vi "TrioMotion Controller.vi"(10 "Notifiers":T2, 11 "Channel in":T1) -> (3 "channel out":T1)   [LabVIEW 2020, in "TrioMotion Controller.lvlib"]
uses:
  TrioMotion Controller.lvlib
  <extravilib>/ChannelInstances/Messenger-t'Message Queue.lvlib-Message Cluster.ctl'/))Channel.ctl
  support/Message Queue/Message Cluster.ctl
  support/Notifiers/Notifiers.ctl
  TrioData.ctl
  Connection Type.ctl
  Axis Parameters.ctl
  controls/MHL Data.ctl
  controls/MHL UI Data.ctl
  controls/MHL Status.ctl
  controls/MHL References.ctl
  controls/MHL Configuration.ctl
  support/SR-Test Med System Globals.vi
  <vilib>/Utility/error.llb/Error Cluster From Error Code.vi
  <vilib>/ErrorRing/Error Ring.xnode
  support/Message Queue/Message Queue.lvlib
  <extravilib>/ChannelInstances/Messenger-t'Message Queue.lvlib-Message Cluster.ctl'.lvlib
panel:
  in  "TrioPC":refnum<k7>(container)
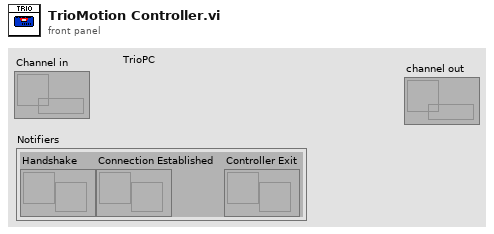
[diagram p1: front panel]
types:
  T1 = typedef "Messenger-t'Message Queue.lvlib-Message Cluster.ctl'.lvlib/))Channel.ctl" = refnum<queue>
  T2 = typedef "Notifiers.ctl" = cluster{"Handshake":refnum<notifier>, "Connection Established":refnum<notifier>, "Controller Exit":refnum<notifier>}
  T3 = typedef "TrioMotion Controller.lvlib/TrioData.ctl" = cluster{"Connected":bool, "Connection Method":T4, "Product Name":string, " Version":string, "Controller Type":string, "SerialCommPort":fxp<+,3,3>, "Programs List":string[], "X Axis Parameters":T5, "A Axis Parameters":T5}
  T4 = typedef "TrioMotion Controller.lvlib/Connection Type.ctl" = enum16{"USB", "Serial", "Ethernet", "PCI", "Path", "No connection"}
  T5 = typedef "TrioMotion Controller.lvlib/Axis Parameters.ctl" = cluster{"ATYPE":dbl, "P_GAIN":dbl, "I_GAIN":dbl, "D_GAIN":dbl, "0V_GAIN":dbl, "VFF_GAIN":dbl, "UNITS":dbl, "SPEED":dbl, "ACCEL":dbl, "DECEL":dbl, "CREEP":dbl, "JOGSPEED":dbl, "FE_LIMIT":dbl, "DAC":dbl, "SERVO":dbl, "REP_DIST":dbl, "FWD_IN":dbl, "REV_IN":dbl, "DATUM_IN":dbl, "FH_IN":dbl, "FS_LIMIT":dbl, "RS_LIMIT":dbl, "MTYPE":dbl, "NTYPE":dbl, "MPOS":dbl, "FE":dbl, "AXISSTATUS":dbl, "VPSPEED":dbl}
  T6 = enum16{"open", "replace", "create", "open or create", "replace or create", "replace or create with confirmation"}
  T7 = typedef "MHL Data.ctl" = cluster{"MHL UI Data":T8, "MHL References":T10, "MHL Configuration":T11}
  T8 = typedef "MHL UI Data.ctl" = cluster{"Status":string, "Connection Type":T4, "Connected to Controller":bool, "Axes Enabled":bool, "Jogging Enabled":bool, "X Axis MPOS":dbl, "A Axis MPOS":dbl, "X Axis SPEED":dbl, "A Axis SPEED":dbl, "Plot Laser Data":bool, "MHL Status":T9}
  T9 = typedef "MHL Status.ctl" = enum16{"Disconnected", "Connecting", "Connected", "Axes Enabled", "Machine Running", "Shutdown"}
  T10 = typedef "MHL References.ctl" = cluster{"Connect to Controller Ref":refnum<vi>, "Connection Type Ref":refnum<vi>, "Set Parameters Ref":refnum<vi>, "Enable Axes Ref":refnum<vi>, "Home Axes Ref":refnum<vi>}
  T11 = typedef "MHL Configuration.ctl" = cluster{"Fuel Control Valve Maximum":dbl, "Fuel Control Valve Minimum":dbl}
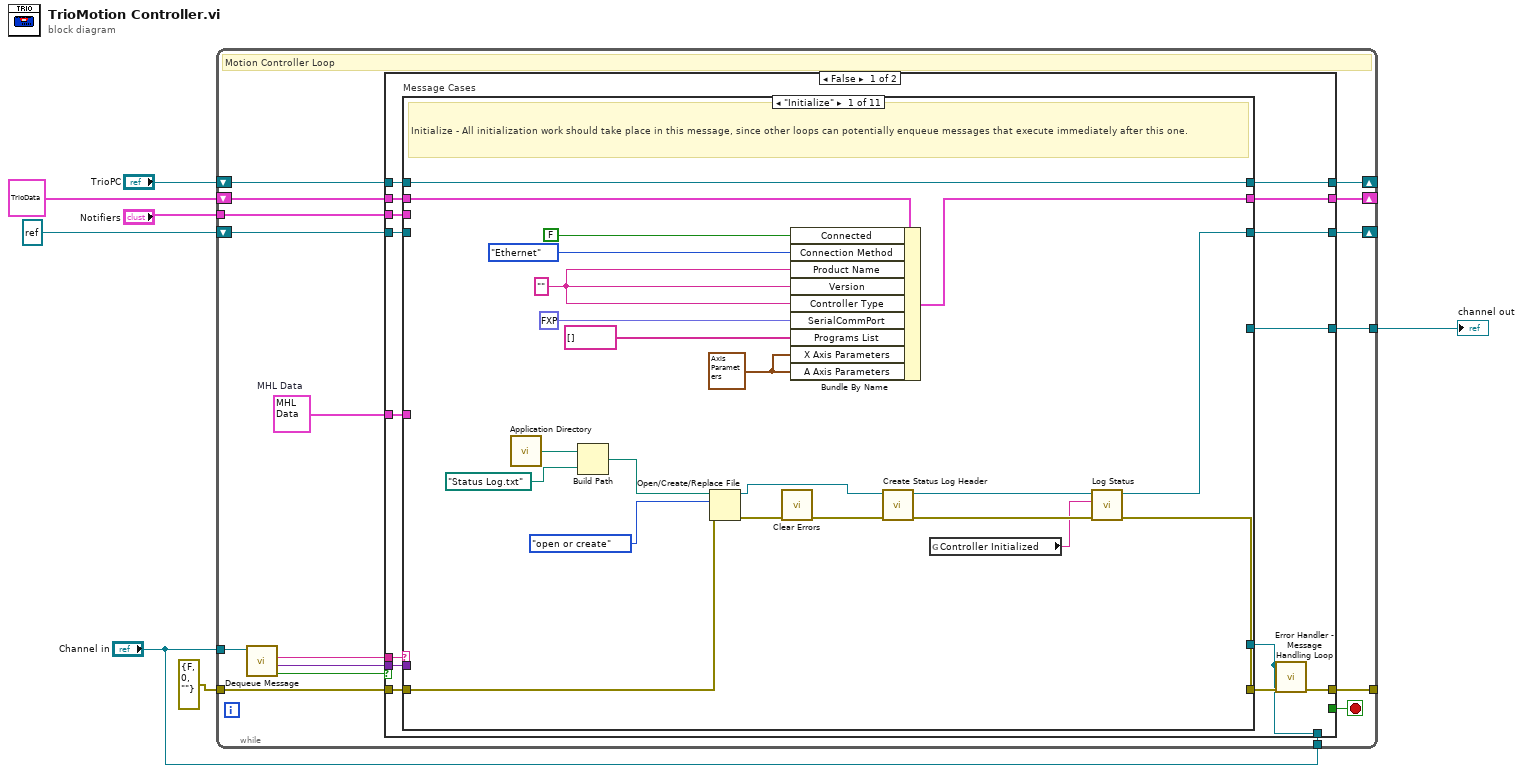
[diagram p0: block diagram]
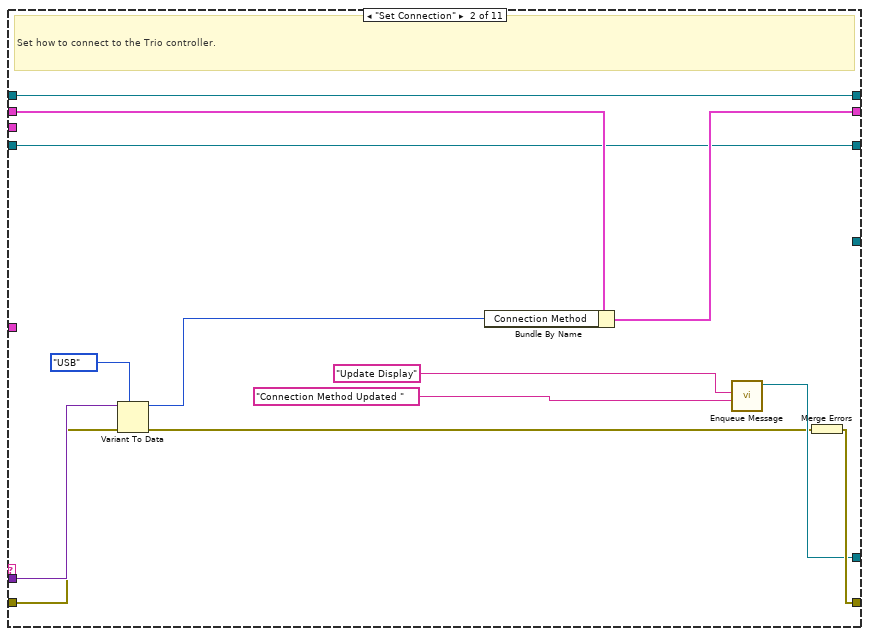
[diagram p2: hidden frame]
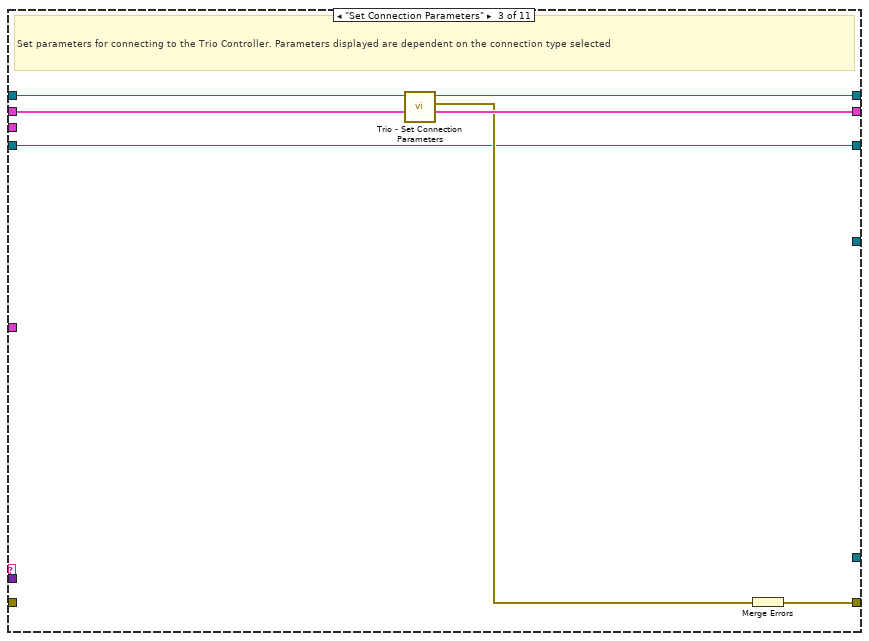
[diagram p3: hidden frame]
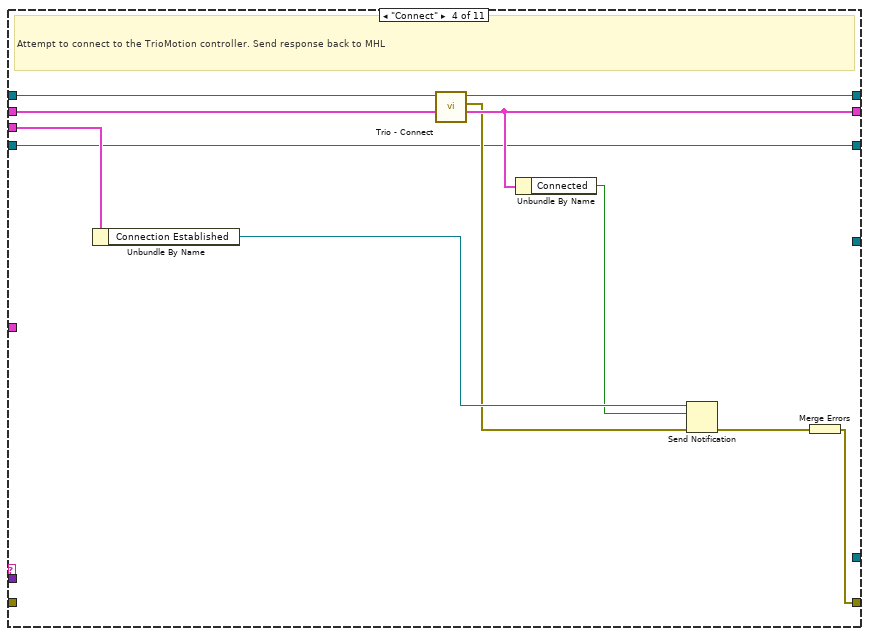
[diagram p4: hidden frame]
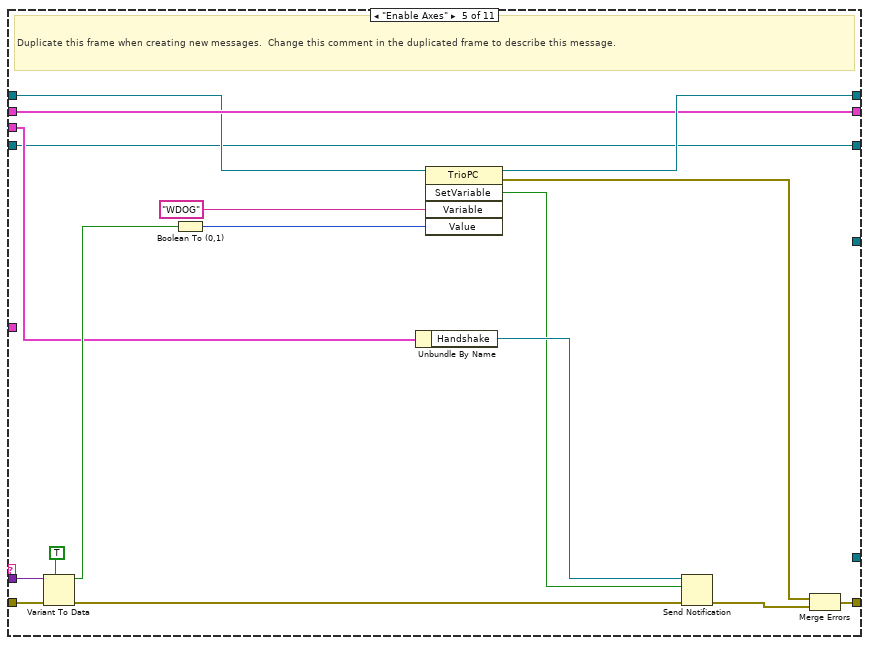
[diagram p5: hidden frame]
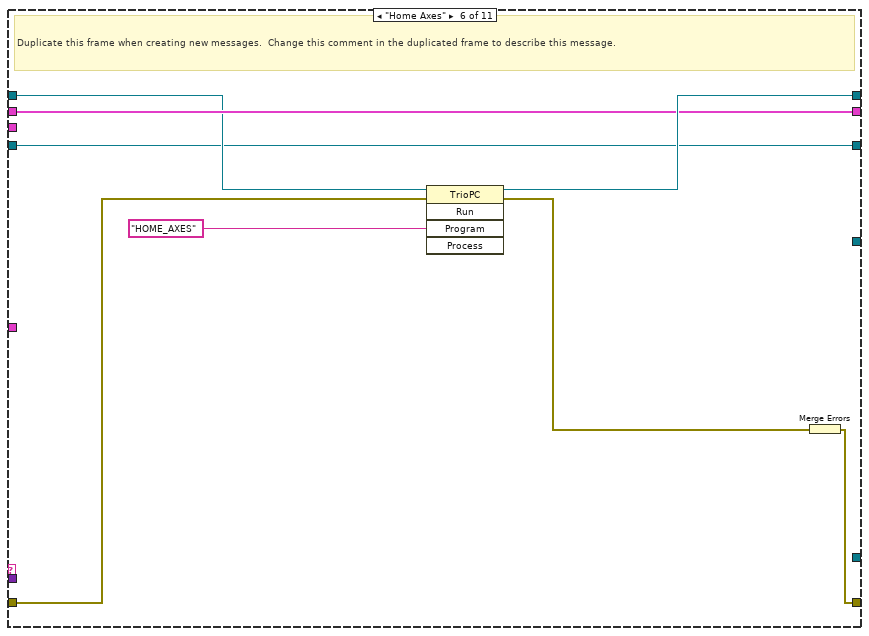
[diagram p6: hidden frame]
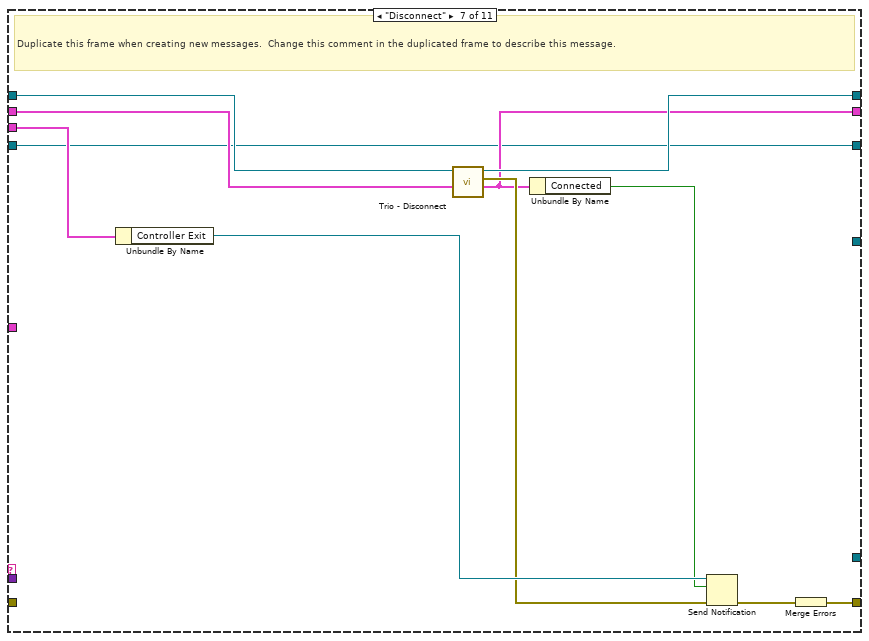
[diagram p7: hidden frame]
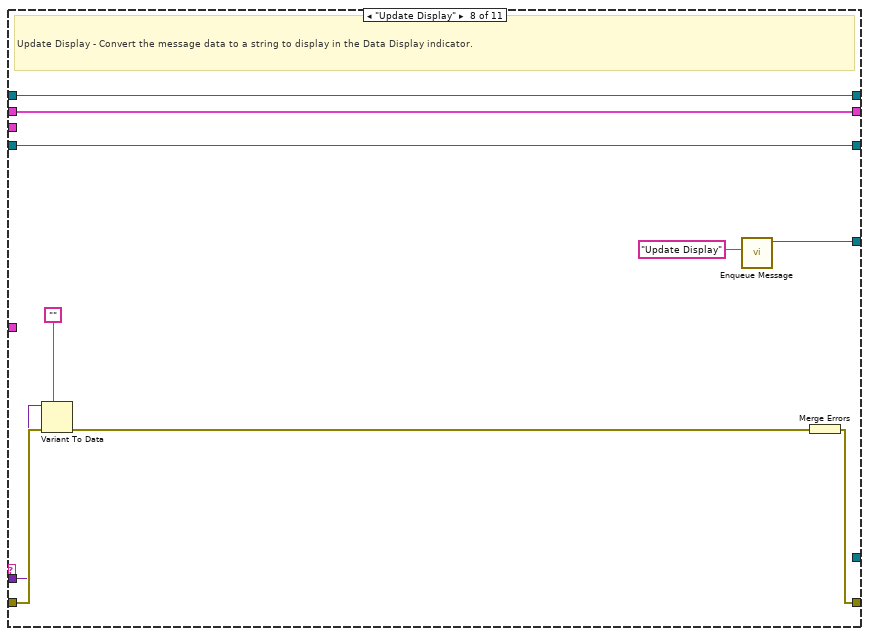
[diagram p8: hidden frame]
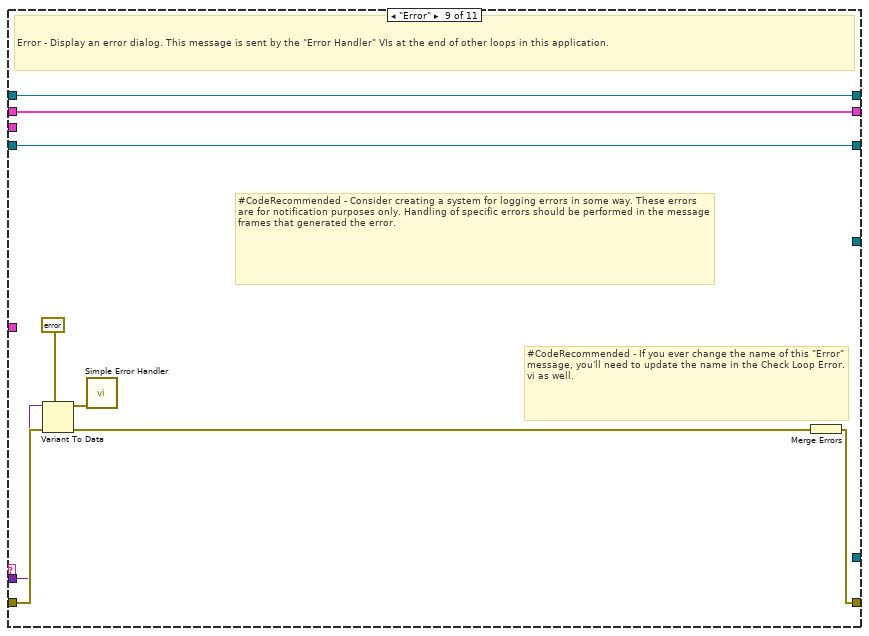
[diagram p9: hidden frame]
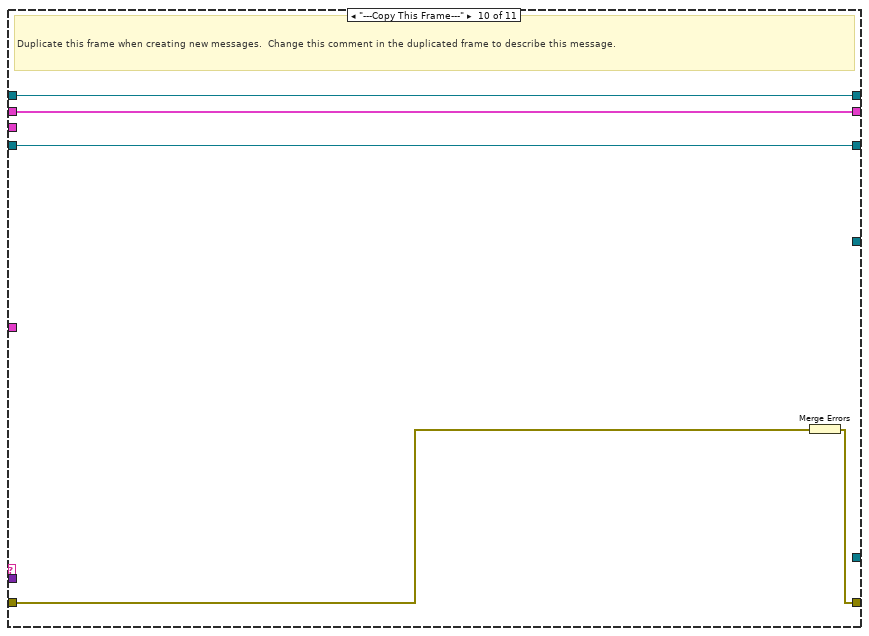
[diagram p10: hidden frame]
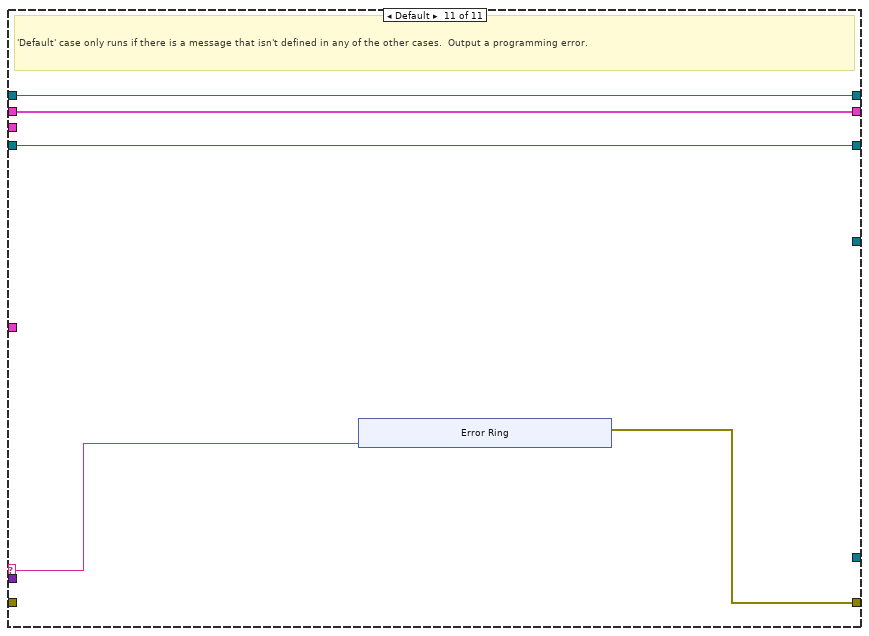
[diagram p11: hidden frame]
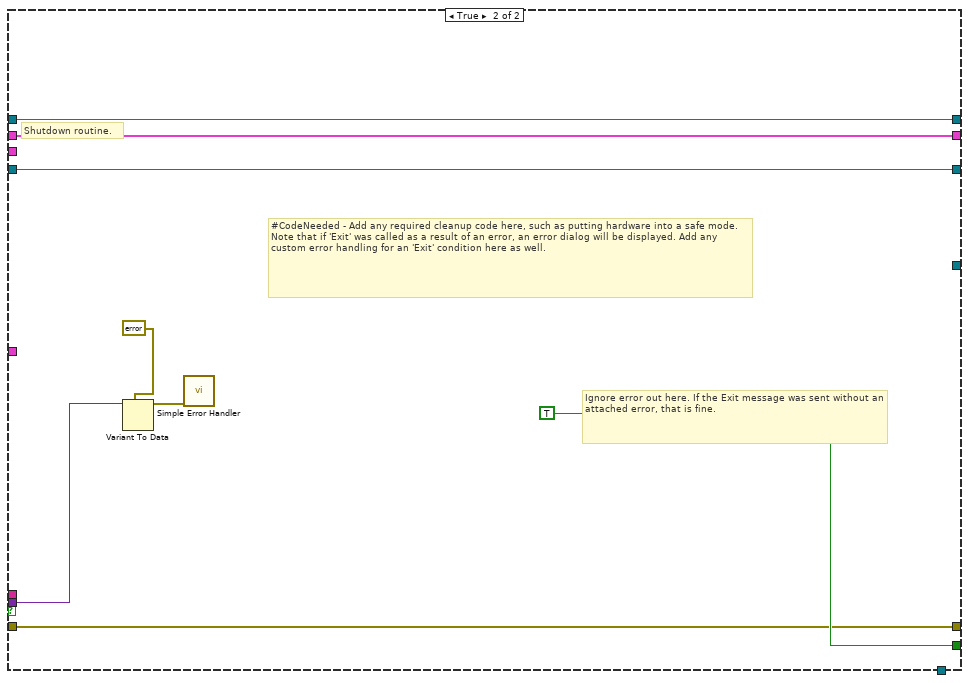
[diagram p12: hidden frame]
diagram:
  n1 = while {
    shift-right: [w23] -> _
    shift-left: T3 {"Connected"=FALSE, "Connection Method"=enum."USB", "Product Name"="", " Version"="", "Controller Type"="", "SerialCommPort"=0.0, "Programs List"=[], "X Axis Parameters"={"ATYPE"=0.0, "P_GAIN"=0.0, "I_GAIN"=0.0, "D_GAIN"=0.0, "0V_GAIN"=0.0, "VFF_GAIN"=0.0, "UNITS"=0.0, "SPEED"=0.0, "ACCEL"=0.0, "DECEL"=0.0, "CREEP"=0.0, "JOGSPEED"=0.0, "FE_LIMIT"=0.0, "DAC"=0.0, "SERVO"=0.0, "REP_DIST"=0.0, "FWD_IN"=0.0, "REV_IN"=0.0, "DATUM_IN"=0.0, "FH_IN"=0.0, "FS_LIMIT"=0.0, "RS_LIMIT"=0.0, "MTYPE"=0.0, "NTYPE"=0.0, "MPOS"=0.0, "FE"=0.0, "AXISSTATUS"=0.0, "VPSPEED"=0.0}, "A Axis Parameters"={"ATYPE"=0.0, "P_GAIN"=0.0, "I_GAIN"=0.0, "D_GAIN"=0.0, "0V_GAIN"=0.0, "VFF_GAIN"=0.0, "UNITS"=0.0, "SPEED"=0.0, "ACCEL"=0.0, "DECEL"=0.0, "CREEP"=0.0, "JOGSPEED"=0.0, "FE_LIMIT"=0.0, "DAC"=0.0, "SERVO"=0.0, "REP_DIST"=0.0, "FWD_IN"=0.0, "REV_IN"=0.0, "DATUM_IN"=0.0, "FH_IN"=0.0, "FS_LIMIT"=0.0, "RS_LIMIT"=0.0, "MTYPE"=0.0, "NTYPE"=0.0, "MPOS"=0.0, "FE"=0.0, "AXISSTATUS"=0.0, "VPSPEED"=0.0}} ("TrioData") -> [w24]
    tunnel: [w21] -> _
    tunnel: "Channel in" -> [w18]
    tunnel: errorcluster {"status"=FALSE, "code"=0, "source"=""} ("error IO") -> [w20]
    tunnel: "Channel in" -> [w19]
    shift-right: [w13] -> _
    shift-left: "TrioPC" -> [w14]
    tunnel: "Notifiers" -> [w12]
    tunnel: [w11] -> w3
    shift-right: [w8] -> _
    shift-left: refnum<file> refnum ("Log File Refnum Out") -> [w9]
    stop <- w22 stop-if-true
    w10 = T7 {"MHL UI Data"={"Status"="", "Connection Type"=enum."Ethernet", "Connected to Controller"=FALSE, "Axes Enabled"=FALSE, "Jogging Enabled"=FALSE, "X Axis MPOS"=0.0, "A Axis MPOS"=0.0, "X Axis SPEED"=0.0, "A Axis SPEED"=0.0, "Plot Laser Data"=FALSE, "MHL Status"=enum."Disconnected"}, "MHL References"={"Connect to Controller Ref"=refnum, "Connection Type Ref"=refnum, "Set Parameters Ref"=refnum, "Enable Axes Ref"=refnum, "Home Axes Ref"=refnum}, "MHL Configuration"={"Fuel Control Valve Maximum"=0.0, "Fuel Control Valve Minimum"=0.0}}  # MHL Data
    # "Motion Controller Loop"
    n2 = call "Dequeue Message.vi"("channel"=w18) -> ("channel aborted"=w15:bool, "message data"=w16:variant, "message"=w17:string)  [unwired: 8 in]
    n3 = case shown="False" w15 {
      tunnel: w24 -> [w39 w170]
      tunnel: [w38 w170] -> w23
      tunnel: [_ TRUE] -> w22
      tunnel: [w37 w171] -> w21
      tunnel: w17 -> [w35 _]
      tunnel: w16 -> [w34 w167]
      tunnel: w20 -> [w33 w171]
      tunnel: [w32 _] -> w19
      tunnel: w14 -> [w31 w166]
      tunnel: [w30 w166] -> w13
      tunnel: w12 -> [w29 _]
      tunnel: [w28 _] -> w11
      tunnel: w10 -> [w27 _]
      tunnel: w9 -> [w26 w165]
      tunnel: [w25 w165] -> w8
      frame False {
        n4 = case "Message Cases" shown="\"Initialize\"" w35 {
          selector: w35 -> [_ _ _ _ _ _ _ _ _ _ w155]
          tunnel: w33 -> [w47 w66 _ _ w103 w111 _ w136 w147 w152 _]
          tunnel: [w40 w74 w81 w92 w109 w117 w128 w137 w141 w150 w156] -> w36
          tunnel: w39 -> [w61 w69 w80 w89 w107 w115 w125 w138 w146 w151 w157]
          tunnel: [w60 w67 w79 w88 w107 w115 w121 w138 w146 w151 w157] -> w38
          tunnel: w34 -> [_ w68 _ _ w102 _ _ w135 w145 _ _]
          tunnel: [_ w73 _ _ _ _ _ _ _ _ _] -> w32
          tunnel: w31 -> [w56 w64 w78 w91 w106 w114 w127 w132 w140 w149 w154]
          tunnel: [w56 w64 w77 w90 w108 w116 w126 w132 w140 w149 w154] -> w30
          tunnel: w29 -> [_ _ _ w87 w99 _ w123 _ _ _ _]
          tunnel: [_ _ _ _ _ _ _ w131 _ _ _] -> w28
          tunnel: w27 -> [_ _ _ _ _ _ _ _ _ _ _]
          tunnel: w26 -> [_ w62 w75 w82 w93 w110 w118 w129 w139 w148 w153]
          tunnel: [w41 w62 w75 w82 w93 w110 w118 w129 w139 w148 w153] -> w25
          frame "Initialize" {
            w53 = T5 {"ATYPE"=0.0, "P_GAIN"=0.0, "I_GAIN"=0.0, "D_GAIN"=0.0, "0V_GAIN"=0.0, "VFF_GAIN"=0.0, "UNITS"=0.0, "SPEED"=0.0, "ACCEL"=0.0, "DECEL"=0.0, "CREEP"=0.0, "JOGSPEED"=0.0, "FE_LIMIT"=0.0, "DAC"=0.0, "SERVO"=0.0, "REP_DIST"=0.0, "FWD_IN"=0.0, "REV_IN"=0.0, "DATUM_IN"=0.0, "FH_IN"=0.0, "FS_LIMIT"=0.0, "RS_LIMIT"=0.0, "MTYPE"=0.0, "NTYPE"=0.0, "MPOS"=0.0, "FE"=0.0, "AXISSTATUS"=0.0, "VPSPEED"=0.0} ("X Axis Parameters")
            w55 = "" ("Product Name")
            # "Initialize - All initialization work should take place in this message, since other loops can potentially enqueue messages that execute immediately after this one."
            n5 = call <vilib>:"Application Directory.vi"() -> ("Application Directory"=w52:path)
            n6 = Build Path(base path=w52, name or relative path=path "Status Log.txt") -> (appended path=w50:path)
            n7 = Open/Create/Replace File(file path (use dialog)=w50, error in=w47, operation (0:open)=T6."open or create") -> (refnum out=w45:refnum<file>, error out=w48:errorcluster)  [unwired: 3 in, 1 out]
            n8 = call <vilib>:"Clear Errors.vi"("error in (no error)"=w48) -> ("error out"=w46:errorcluster)  [unwired: 5 in, 1 out]
            n9 = Bundle By Name(cluster=w61, "Connected"=FALSE, "Connection Method"=Connection_Type."Ethernet", "Product Name"=w55, "Version"=w55, "Controller Type"=w55, "SerialCommPort"=fxp<+,3,3> 0.0, "Programs List"=string[] [], "X Axis Parameters"=w53, "A Axis Parameters"=w53) -> (w60:T3)
            n10 = call "Create Status Log Header.vi"("error in"=w46, "Log File Refnum in"=w45) -> ("error out"=w44:errorcluster, "Log File Refnum out"=w43:refnum<file>)  [unwired: 8 in]
            n11 = global read "SR-Test Med System Globals.vi" "Controller Initialized"() -> (w42:string)
            n12 = call "Log Status.vi"("error in"=w44, "Event String"=w42, "Log File Refnum In"=w43) -> ("error out"=w40:errorcluster, "Log File Refnum Out"=w41:refnum<file>)  [unwired: 7 in]
          }
          frame "Set Connection" {
            # "Set how to connect to the Trio controller."
            n13 = Variant To Data(error in=w66, type=Connection_Type."USB" ("Connection Method"), Variant=w68) -> (data=w70:T4, error out=w65:errorcluster)
            n14 = Bundle By Name(cluster=w69, "Connection Method"=w70) -> (w67:T3)
            n15 = call "Enqueue Message.vi"("data (empty)"="Connection Method Updated " ("\"Do Something\" button pressed"), "message"="Update Display" ("Message")) -> ("channel"=w73:T1)  [unwired: 9 in]
            n16 = Merge Errors(w65) -> (w74:errorcluster)
          }
          frame "Set Connection Parameters" {
            # "Set parameters for connecting to the Trio Controller. Parameters displayed are dependent on the connection type selected"
            n17 = call "Trio - Set Connection Parameters.vi"("TrioData In"=w80, "TrioControl Refnum in"=w78) -> ("TrioData Out"=w79:T3, "error out"=w76:errorcluster, "TrioControl Refnum Out"=w77:refnum<k7>)  [unwired: 7 in]
            n18 = Merge Errors(w76) -> (w81:errorcluster)
          }
          frame "Connect" {
            # "Attempt to connect to the TrioMotion controller. Send response back to MHL"
            n19 = Unbundle By Name(w87) -> ("Connection Established"=w86:refnum<notifier>)
            n20 = call "Trio - Connect.vi"("TrioData In"=w89, "Trio Reference In"=w91) -> ("TrioData Out"=w88:T3, "error out"=w83:errorcluster, "Trio Reference Out"=w90:refnum<k7>)  [unwired: 7 in]
            n21 = Unbundle By Name(w88) -> ("Connected"=w85:bool)
            n22 = Send Notification(notification=w85, notifier=w86, error in (no error)=w83) -> (error out=w84:errorcluster)  [unwired: 1 out]
            n23 = Merge Errors(w84) -> (w92:errorcluster)
          }
          frame "Enable Axes" {
            # "Duplicate this frame when creating new messages.  Change this comment in the duplicated frame to describe this message."
            n24 = Variant To Data(error in=w103, type=TRUE, Variant=w102) -> (data=w101:bool, error out=w94:errorcluster)
            n25 = Boolean To (0,1)(Boolean=w101) -> (0, 1=w100:i16)
            n26 = Unbundle By Name(w99) -> ("Handshake"=w98:refnum<notifier>)
            n27 = invoke class="TrioPC" method="SetVariable"(reference=w106, "Variable"="WDOG", "Value"=w100) -> (reference out=w108:refnum<k7>, error out=w95:errorcluster, "SetVariable"=w97:bool)  [unwired: 2 in, 2 out]
            n28 = Send Notification(notification=w97, notifier=w98, error in (no error)=w94) -> (error out=w96:errorcluster)  [unwired: 1 out]
            n29 = Merge Errors(w95, w96) -> (w109:errorcluster)
          }
          frame "Home Axes" {
            # "Duplicate this frame when creating new messages.  Change this comment in the duplicated frame to describe this message."
            n30 = invoke class="TrioPC" method="Run"(reference=w114, error in=w111, "Program"="HOME_AXES" ("Variable")) -> (reference out=w116:refnum<k7>, error out=w113:errorcluster)  [unwired: 2 in, 3 out]
            n31 = Merge Errors(w113) -> (w117:errorcluster)
          }
          frame "Disconnect" {
            # "Duplicate this frame when creating new messages.  Change this comment in the duplicated frame to describe this message."
            n32 = Unbundle By Name(w123) -> ("Controller Exit"=w124:refnum<notifier>)
            n33 = call "Trio - Disconnect.vi"("TrioData In"=w125, "Trio Reference In"=w127) -> ("TrioData Out"=w121:T3, "error out"=w122:errorcluster, "Trio Reference Out"=w126:refnum<k7>)  [unwired: 7 in]
            n34 = Unbundle By Name(w121) -> ("Connected"=w120:bool)
            n35 = Send Notification(notification=w120, notifier=w124, error in (no error)=w122) -> (error out=w119:errorcluster)  [unwired: 1 out]
            n36 = Merge Errors(w119) -> (w128:errorcluster)
          }
          frame "Update Display" {
            # "Update Display - Convert the message data to a string to display in the Data Display indicator."
            n37 = Variant To Data(error in=w136, type="", Variant=w135) -> (error out=w133:errorcluster)  [unwired: 1 out]
            n38 = call "Enqueue Message.vi"("message"="Update Display") -> ("channel"=w131:T1)  [unwired: 10 in]
            n39 = Merge Errors(w133) -> (w137:errorcluster)
          }
          frame "Error" {
            # "#CodeRecommended - If you ever change the name of this \"Error\" message, you'll need to update the name in the Check Loop Error.vi as well."
            # "#CodeRecommended - Consider creating a system for logging errors in some way. These errors are for notification purposes only. Handling of specific errors should be performed in the message frames that generated the error."
            # "Error - Display an error dialog. This message is sent by the \"Error Handler\" VIs at the end of other loops in this application."
            n40 = Variant To Data(error in=w147, type=errorcluster {"status"=FALSE, "code"=0, "source"=""} ("error constant"), Variant=w145) -> (data=w143:errorcluster, error out=w142:errorcluster)
            n41 = call <vilib>:"Simple Error Handler.vi"("error in (no error)"=w143) -> ()  [unwired: 4 in, 5 out]
            n42 = Merge Errors(w142) -> (w141:errorcluster)
          }
          frame "---Copy This Frame---" {
            # "Duplicate this frame when creating new messages.  Change this comment in the duplicated frame to describe this message."
            n43 = Merge Errors(w152) -> (w150:errorcluster)
          }
          frame Default {
            # "'Default' case only runs if there is a message that isn't defined in any of the other cases.  Output a programming error."
            n44 = xnode "Error Ring"("parameter 0"=w155) -> ("error out"=w156:errorcluster)
          }
        }
        n45 = call "Error Handler - Message Handling Loop.vi"("channel"=w32, "error in (no error)"=w36) -> ("dup error in"=w37:errorcluster)  [unwired: 9 in]
      }
      frame True {
        # "Ignore error out here. If the Exit message was sent without an attached error, that is fine."
        # "#CodeNeeded - Add any required cleanup code here, such as putting hardware into a safe mode. Note that if 'Exit' was called as a result of an error, an error dialog will be displayed. Add any custom error handling for an 'Exit' condition here as well."
        # "Shutdown routine."
        n46 = Variant To Data(type=errorcluster {"status"=FALSE, "code"=0, "source"=""} ("error constant"), Variant=w167) -> (data=w168:errorcluster)  [unwired: 1 in, 1 out]
        n47 = call <vilib>:"Simple Error Handler.vi"("error in (no error)"=w168) -> ()  [unwired: 4 in, 5 out]
      }
    }
  }
  "channel out" <- w3
